vi "Launcher.vi"   [LabVIEW 2020]
uses:
  Spanish Picker/Spanish Picker.lvclass
  D:/Storage/Source Code/Clase AF/ClaseAF/05 AF Camera/Products Picker/Products Picker.lvclass
  English Picker/English Picker/English Picker.lvclass
  Products Picker/Products Picker.lvclass
  C:/Program Files (x86)/National Instruments/LabVIEW 2020/vi.lib/ActorFramework/Actor/Actor.lvclass
  <vilib>/ActorFramework/Actor/Actor.lvclass
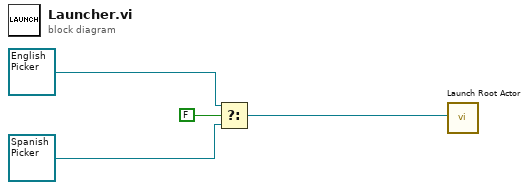
[diagram p0: block diagram]
diagram:
  n1 = Select(t=refnum<class "English Picker.lvclass"> refnum ("English Picker.lvlib:English Picker.lvclass"), s=FALSE, f=refnum<class "Spanish Picker.lvclass"> refnum ("Spanish Picker.lvlib:Spanish Picker.lvclass")) -> (s? t:f=w2:refnum<class "Products Picker.lvclass">)
  n2 = call <vilib>:"Launch Root Actor.vi"("Actor"=w2) -> ()  [unwired: 9 in, 2 out]
